vi "setUp.vi"(8 "error in (no error)":errorcluster, 11 "reference in":refnum<class "Single Core Simple Loopback.lvclass">) -> (0 "error out":errorcluster, 3 "reference out":refnum<class "Single Core Simple Loopback.lvclass">)   [LabVIEW 2020, in "Single Core Simple Loopback.lvclass"]
doc: "setUp runs prior to the test method during test execution. Use this method to initialize any object data required by your tests."
uses:
  Single Core Simple Loopback.lvclass
  C:/Program Files (x86)/National Instruments/LabVIEW 2020/vi.lib/addons/_JKI Toolkits/VI Tester/TestCase.llb/TestCase.lvclass
  <vilib>/addons/_JKI Toolkits/VI Tester/TestCase.llb/TestCase.lvclass
  C:/Users/nitest/Desktop/Git 2020/niveristand-custom-device-testing-tools/VeriStandTestCase/VeriStandTestCase.lvclass
  C:/Users/nitest/Desktop/Git 2020/niveristand-ballard-arinc429-custom-device/Source/Custom Device Support/Tests/System/Single Core (P2--P3) Simple Loopback/Single Core Simple Loopback.lvclass
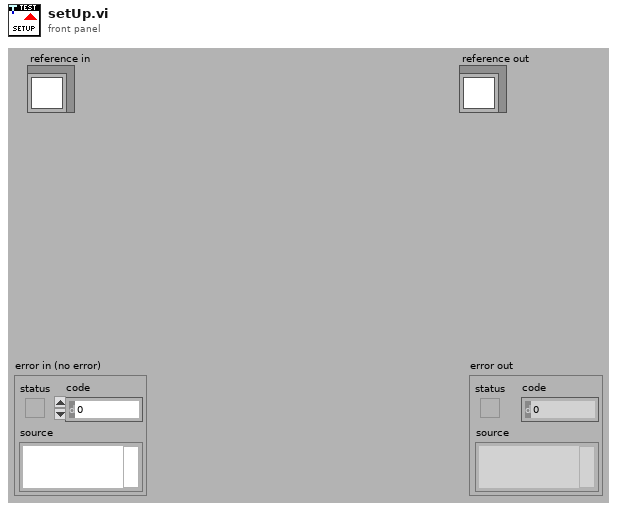
[diagram p1: front panel]
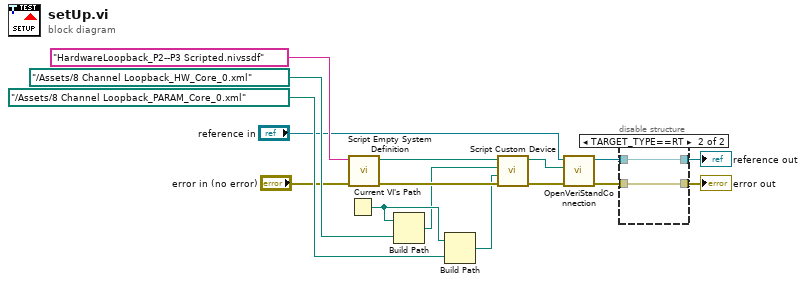
[diagram p0: block diagram]
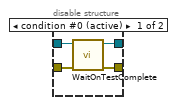
[diagram p2: hidden frame]
diagram:
  n1 = Current VI's Path() -> (path=w12:path)
  n2 = call "Script Empty System Definition.vi"("error in"="error in (no error)", "System Definition Name"="HardwareLoopback_P2--P3 Scripted.nivssdf" ("Channel")) -> ("error out"=w14:errorcluster, "System Definition Path"=w13:path)  [unwired: 8 in]
  n3 = Build Path(base path=w12, name or relative path=path "../Assets/8 Channel Loopback_HW_Core_0.xml" ("Hardware File Path")) -> (appended path=w11:path)
  n4 = Build Path(base path=w12, name or relative path=path "../Assets/8 Channel Loopback_PARAM_Core_0.xml" ("Hardware File Path")) -> (appended path=w10:path)
  n5 = call "Script Custom Device.vi"("error in"=w14, "Parameter File Path"=w10, "Hardware File Path"=w11, "System Definition File Path In"=w13) -> ("error out"=w1:errorcluster, "System Definition File Path Out"=w2:path)  [unwired: 6 in]
  n6 = call-dynamic "OpenVeriStandConnection.vi"("error in (no error)"=w1, "System Definition File"=w2, "VeriStand Test Case in"="reference in") -> ("error out"=w5:errorcluster, "VeriStand Test Case out"=w4:refnum<class "Single Core Simple Loopback.lvclass">)  [unwired: 6 in, 1 out]
  n7 = disable-structure shown="TARGET_TYPE==RT" {
    disable-tunnel: w5 -> [w20 w21]
    disable-tunnel: [w19 w21] -> w16
    disable-tunnel: [w18 w22] -> w15
    disable-tunnel: w4 -> [w17 w22]
    frame condition #0 (active) {
      n8 = call <vilib>:"WaitOnTestComplete.vi"("error in (no error)"=w20, "TestCase in"=w17) -> ("error out"=w19:errorcluster, "TestCase out"=w18:refnum<class "Single Core Simple Loopback.lvclass">)  [unwired: 8 in]
    }
    frame condition #1 {
    }
  }
  "error out" <- w16
  "reference out" <- w15
